vi "ReadDblData.vi"(8 "Error In":errorcluster caption="エラー入力", 10 "データ":T2, 11 "refnum":T1) -> (0 "Error Out":errorcluster caption="エラー出力", 2 "数値":dbl, 3 "refnum out":T1 caption="refnum出力")   [LabVIEW 2015]
doc: "iniファイルからDBLデータを読み込みます。"
uses:
  <vilib>/Utility/config.llb/Config Data RefNum.ctl
  <vilib>/Utility/config.llb/Read Key (Double).vi
  <vilib>/Utility/config.llb/Write Key (Double).vi
  <vilib>/Utility/config.llb/NI_LVConfig.lvlib
panel:
  # "■IniファイルからDBLデータを読込む"
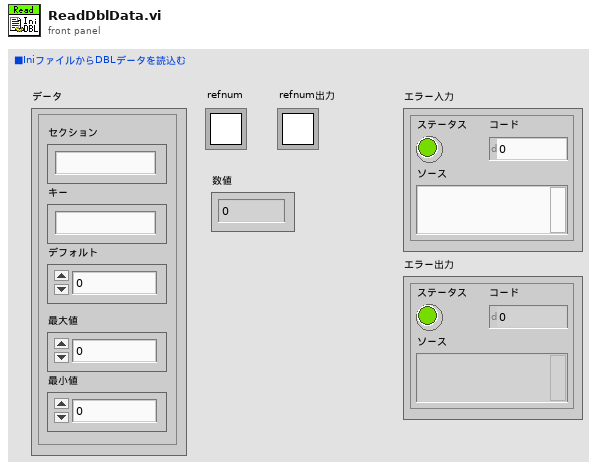
[diagram p1: front panel]
types:
  T1 = typedef "NI_LVConfig.lvlib/Config Data RefNum.ctl" = refnum<k1>
  T2 = cluster{"セクション":string, "キー":string, "デフォルト":dbl, "最大値":dbl, "最小値":dbl}
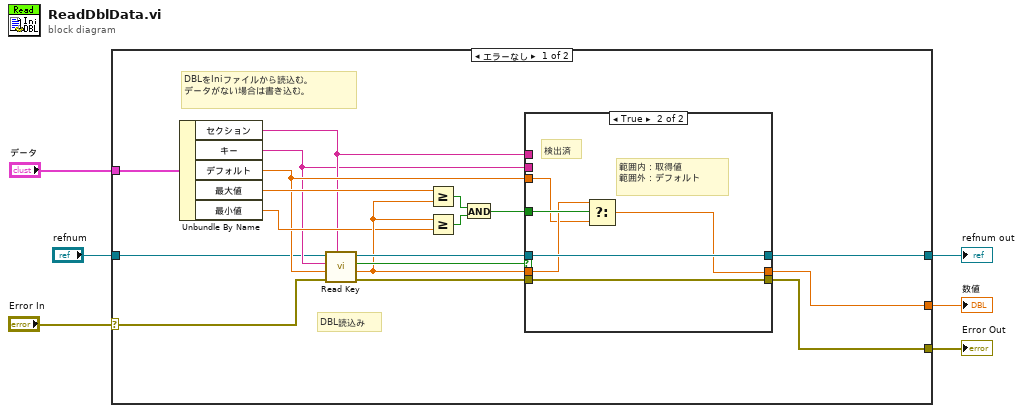
[diagram p0: block diagram]
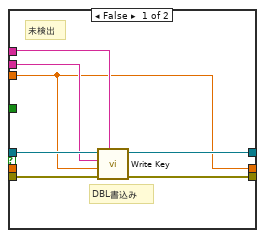
[diagram p2: hidden frame]
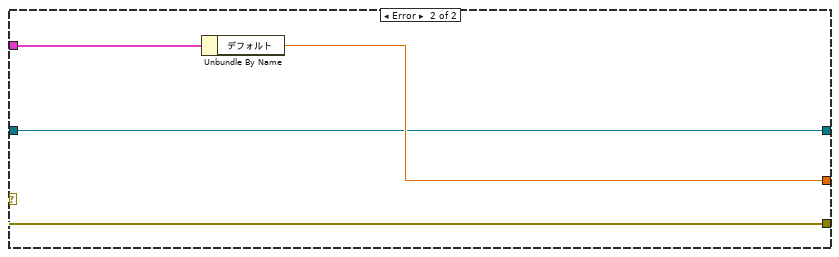
[diagram p3: hidden frame]
diagram:
  n1 = case shown="エラーなし" "Error In" {
    selector: "Error In" -> [w11 w41]
    tunnel: [w12 w41] -> w6
    tunnel: [w10 w39] -> w4
    tunnel: "データ" -> [w9 w40]
    tunnel: [w8 w38] -> w2
    tunnel: "refnum" -> [w7 w38]
    frame No Error {
      # "DBLをIniファイルから読込む。\nデータがない場合は書き込む。"
      # "DBL読込み"
      n2 = Unbundle By Name(w9) -> ("セクション"=w14:string, "キー"=w13:string, "デフォルト"=w15:dbl, "最大値"=w21:dbl, "最小値"=w19:dbl)
      n3 = call-poly <vilib>:"Read Key.vi"("section"=w14, "error in (no error)"=w11, "default value"=w15, "key"=w13, "refnum"=w7) -> ("error out"=w22:errorcluster, "value"=w20:dbl, "found?"=w24:bool, "refnum out"=w23:T1)  [unwired: 3 in]
      n4 = Greater Or Equal?(x=w21, y=w20) -> (x >= y?=w17:bool)
      n5 = Greater Or Equal?(x=w20, y=w19) -> (x >= y?=w18:bool)
      n6 = And(x=w17, y=w18) -> (x .and. y?=w16:bool)
      n7 = case shown="TRUE" w24 {
        tunnel: w23 -> [w31 w37]
        tunnel: [w30 w37] -> w8
        tunnel: w20 -> [_ w34]
        tunnel: [w25 w32] -> w10
        tunnel: w22 -> [w29 w36]
        tunnel: [w28 w36] -> w12
        tunnel: w16 -> [_ w35]
        tunnel: w15 -> [w25 w33]
        tunnel: w14 -> [w27 _]
        tunnel: w13 -> [w26 _]
        frame False {
          # "DBL書込み"
          # "未検出"
          n8 = call-poly <vilib>:"Write Key.vi"("section"=w27, "error in (no error)"=w29, "value"=w25, "key"=w26, "refnum"=w31) -> ("error out"=w28:errorcluster, "refnum out"=w30:T1)  [unwired: 4 in, 1 out]
        }
        frame True {
          # "範囲内：取得値\n範囲外：デフォルト"
          # "検出済"
          n9 = Select(t=w34, s=w35, f=w33) -> (s? t:f=w32:dbl)
        }
      }
    }
    frame Error {
      n10 = Unbundle By Name(w40) -> ("デフォルト"=w39:dbl)
    }
  }
  "Error Out" <- w6
  "数値" <- w4
  "refnum out" <- w2
